vi "DeviceOpen.vi"(8 "error in (no error)":errorcluster, 10 "Delay between send and receive [ms]":i32=100, 11 "GenericDevice in":refnum<class "GenericDevice.lvclass">) -> (0 "error out":errorcluster, 1 "ID":i32, 2 "device is open?":bool, 3 "GenericDevice out":refnum<class "GenericDevice.lvclass">)   [LabVIEW 2023, in "GenericDevice.lvclass"]
uses:
  GenericDevice.lvclass
  GenericDevice.lvclass/GenericDevice.ctl
  08520d01-4428-4ec1-8a34-fbaac9900107.vi
  66473747-6f8a-4511-9a92-322c9b2dd28a.vi
  <vilib>/JDP Science/JSONtext/Variant to JSON Text.vi
  <vilib>/JDP Science/JSONtext/Set Item.vi
  <vilib>/JDP Science/JSONtext/LVClass Serializer/JSONtext LVClass Serializer.lvclass
  <vilib>/IlluminatedG/lv-web-crypto/lv-json/JSON/JSON.lvlib
panel:
  # "Connector Pane"
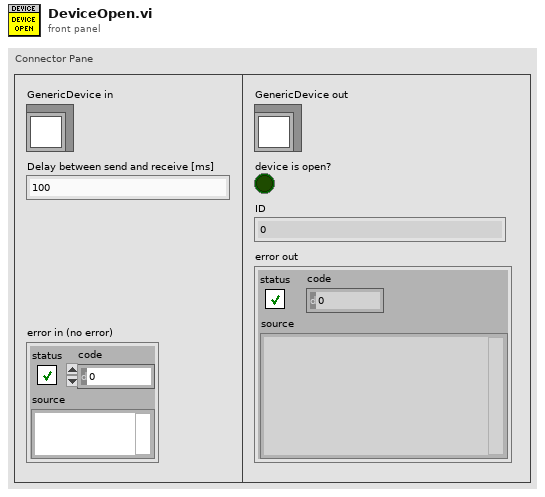
[diagram p1: front panel]
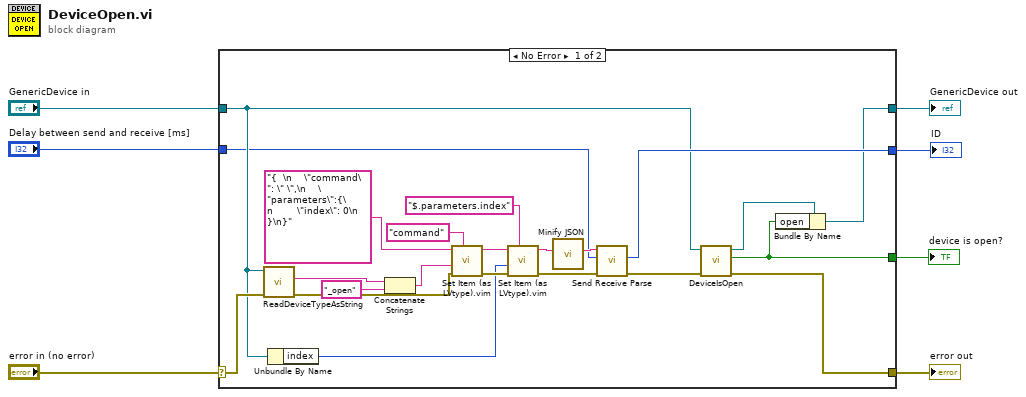
[diagram p0: block diagram]
diagram:
  n1 = case shown="No Error" "error in (no error)" {
    selector: "error in (no error)" -> [w12 w31]
    tunnel: [w16 w31] -> w6
    tunnel: [w14 w30] -> w4
    tunnel: "GenericDevice in" -> [w9 w30]
    tunnel: [w20 _] -> w3
    tunnel: [w13 _] -> w2
    tunnel: "Delay between send and receive [ms]" -> [w8 _]
    frame No Error {
      n2 = call "ReadDeviceTypeAsString.vi"("error in (no error)"=w12, "GenericDevice.lvclass"=w9) -> ("error out"=w11:errorcluster, "String"=w10:string)  [unwired: 7 in, 1 out]
      n3 = Unbundle By Name(w9) -> ("index"=w22:i32)
      n4 = Concatenate Strings(w10, "_open" ("string")) -> (w23:string)
      n5 = call "Set Item (as LVtype).vim"("$Path or Item Name"="command", "error in (no error)"=w11, "Anything"=w23, "JSON"="{  \n    \"command\": \" \",\n    \"parameters\":{\n        \"index\": 0\n    }\n}") -> ("error out"=w27:errorcluster, "<JSON>"=w28:string)  [unwired: 4 in, 1 out]
      n6 = call "Set Item (as LVtype).vim"("$Path or Item Name"="$.parameters.index", "error in (no error)"=w27, "Anything"=w22, "JSON"=w28) -> ("error out"=w21:errorcluster, "<JSON>"=w19:string)  [unwired: 4 in, 1 out]
      n7 = call <vilib>:"Minify JSON.vi"("JSON String"=w19) -> ("Minified JSON"=w18:string)  [unwired: 10 in]
      n8 = call "Send Receive Parse.vi"("error in"=w21, "Delay between send and receive [ms]"=w8, "<JSON>"=w18) -> ("error out"=w17:errorcluster, "ID"=w20:i32)  [unwired: 6 in, 1 out]
      n9 = call-dynamic "DeviceIsOpen.vi"("error in (no error)"=w17, "GenericDevice in"=w9) -> ("error out"=w16:errorcluster, "device is open?"=w13:bool, "GenericDevice out"=w15:refnum<class "GenericDevice.lvclass">)  [unwired: 6 in, 1 out]
      n10 = Bundle By Name(cluster=w15, "open"=w13) -> (w14:refnum<class "GenericDevice.lvclass">)
    }
    frame Error {
    }
  }
  "error out" <- w6
  "GenericDevice out" <- w4
  "ID" <- w3
  "device is open?" <- w2
